vi "Start Controller.vi"(8 "error in (no error)":errorcluster, 10 "Window Handle":i32, 11 "Config File Path":path=path "TestStand.ini") -> (0 "error out":errorcluster, 2 "Path to config file":path, 3 "Controller Queue":refnum<class "Message Enqueuer.lvclass">)   [LabVIEW 2015, in "TestStand API.lvlib"]
uses:
  TestStand API.lvlib
  <vilib>/ActorFramework/Message Enqueuer/Message Enqueuer.lvclass
  <userlib>/Measurement Utility API/Controller API.lvclass
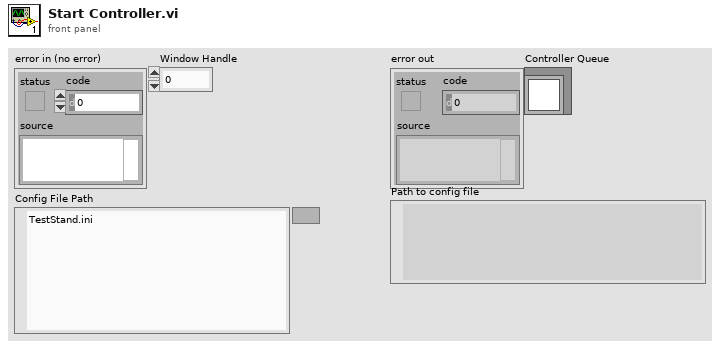
[diagram p1: front panel]
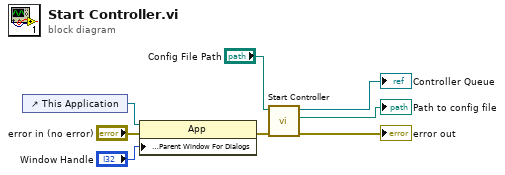
[diagram p0: block diagram]
diagram:
  n1 = control-ref of="This Application"() -> (w3:refnum<vi>)
  n2 = property class="App"(reference=w3, error in="error in (no error)", "Application:Parent Window For Dialogs"="Window Handle") -> (error out=w2:errorcluster)  [unwired: 1 out]
  n3 = call <userlib>:"Start Controller.vi"("error in (no error)"=w2, "Config File Path"="Config File Path") -> ("error out"=→"error out":errorcluster, "Path to config file"=→"Path to config file":path, "Controller Queue"=→"Controller Queue":refnum<class "Message Enqueuer.lvclass">)  [unwired: 7 in]
